vi "Tab Add.vi"(8 "error in (no error)":errorcluster, 10 "Tab Name":string, 11 "VI Refnum":refnum<vi>) -> (0 "error out":errorcluster)   [LabVIEW 2018, in "Tab.lvlib"]
uses:
  Tab.lvlib
  Tab Action.ctl
  Tab Add.ctl
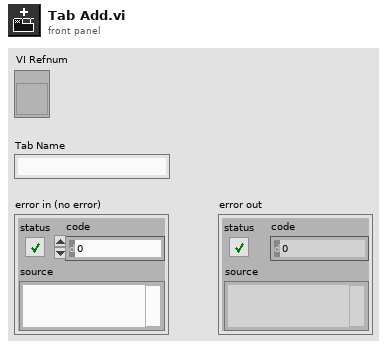
[diagram p1: front panel]
types:
  T1 = typedef "Tab.lvlib/Tab Add.ctl" = cluster{"VI Path":path, "Name":string}
  T2 = typedef "Tab.lvlib/Tab Action.ctl" = enum8{"noop", "new", "init", "close", "start", "render", "tab_add", "tab_change", "tab_hover", "tab_event", "tab_insert", "tab_popout", "tab_close", "theme_change", "resize"}
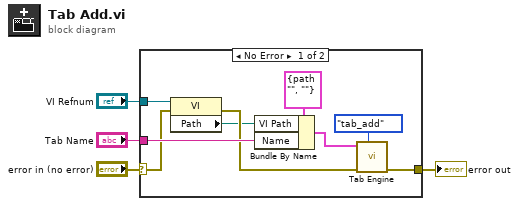
[diagram p0: block diagram]
diagram:
  n1 = case shown="No Error" "error in (no error)" {
    selector: "error in (no error)" -> [w7 w14]
    tunnel: [w12 w14] -> w4
    tunnel: "Tab Name" -> [w10 _]
    tunnel: "VI Refnum" -> [w8 _]
    frame No Error {
      n2 = property class="VI"(reference=w8, error in=w7) -> (error out=w6:errorcluster, "Path"=w5:path)  [unwired: 1 out]
      n3 = Bundle By Name(cluster=T1 {"VI Path"=path "", "Name"=""} ("Tab Add"), "VI Path"=w5, "Name"=w10) -> (w9:T1)
      n4 = call "Tab Engine.vi"("Action"=Tab_Action."tab_add", "error in (no error)"=w6, "Variant in"=w9) -> ("error out"=w12:errorcluster)  [unwired: 7 in, 1 out]
    }
    frame Error {
    }
  }
  "error out" <- w4
